vi "Map Neighbors.vi"(10 "Position":cluster{"Row":i32, "Col":i32}, 11 "Map":T1) -> (2 "Neighbors":cluster{"Row":i32, "Col":i32}[](array[cluster]))   [LabVIEW 2022 SP3, in "AoC22.lvlib"]
uses:
  AoC22.lvlib
  Map.ctl
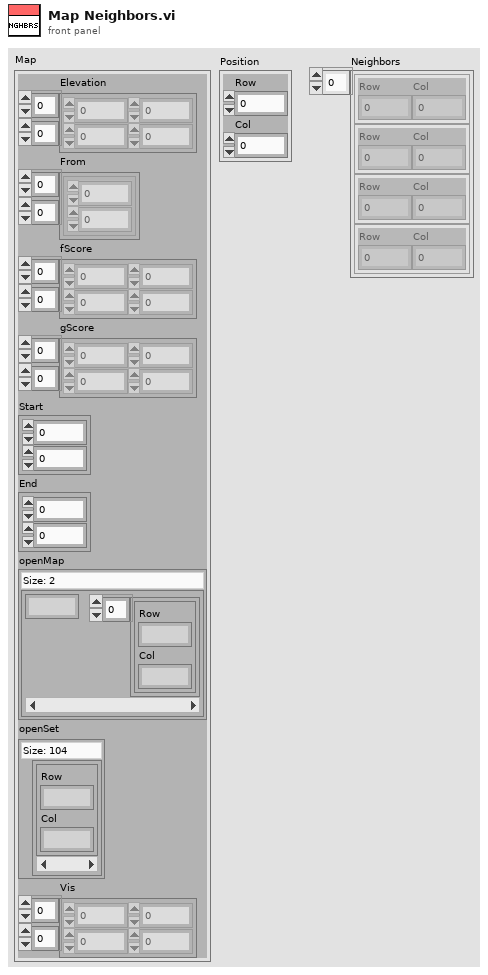
[diagram p1: front panel]
types:
  T1 = typedef "AoC22.lvlib/Map.ctl" = cluster{"Elevation":u8[][], "From":cluster{"Row":i32, "Col":i32}[][], "fScore":i32[][], "gScore":i32[][], "Start":cluster{"Row":i32, "Col":i32}, "End":cluster{"Row":i32, "Col":i32}, "openMap":map{i32, cluster{"Row":i32, "Col":i32}[]}, "openSet":set{cluster{"Row":i32, "Col":i32}}, "Vis":u8[][]}
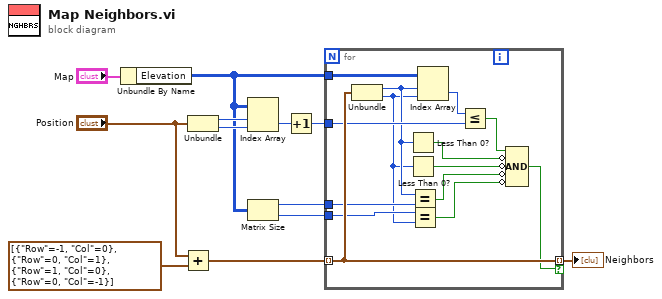
[diagram p0: block diagram]
diagram:
  n1 = Unbundle By Name("Map") -> ("Elevation"=w3:u8[][])
  n2 = Add(x="Position", y=cluster{"Row":i32, "Col":i32}[] [{"Row"=-1, "Col"=0}, {"Row"=0, "Col"=1}, {"Row"=1, "Col"=0}, {"Row"=0, "Col"=-1}] ("Position")) -> (x+y=w10:cluster{"Row":i32, "Col":i32}[])
  n3 = Unbundle("Position") -> ("Row"=w8:i32, "Col"=w7:i32)
  n4 = Index Array(array=w3, index (row)=w8, index (col)=w7) -> (element=w6:u8)
  n5 = Matrix Size(0:w3) -> (1:w2:i32, 2:w1:i32)
  n6 = Increment(x=w6) -> (x+1=w5:u8)
  n7 = for {
    tunnel: w10 -> [w26] mode=indexing
    tunnel: w3 -> [w25]
    tunnel: w5 -> [w24]
    tunnel: [w26] -> w4 mode=indexing if=w13
    tunnel: w2 -> [w22]
    tunnel: w1 -> [w21]
    n8 = Unbundle(w26) -> ("Row"=w20:i32, "Col"=w19:i32)
    n9 = Less Than 0?(x=w20) -> (x < 0?=w16:bool)
    n10 = Less Than 0?(x=w19) -> (x < 0?=w17:bool)
    n11 = Equal?(x=w20, y=w22) -> (x = y?=w15:bool)
    n12 = Equal?(x=w21, y=w19) -> (x = y?=w14:bool)
    n13 = Index Array(array=w25, index (row)=w20, index (col)=w19) -> (element=w23:u8)
    n14 = Less Or Equal?(x=w23, y=w24) -> (x <= y?=w18:bool)
    n15 = Compound Arithmetic op=AND(w18, invert w16, invert w17, invert w15, invert w14) -> (w13:bool)
  }
  "Neighbors" <- w4
